vi "CG_Protokoll.vi"(6 "Aktion":T1, 8 "Pfad":path, 10 "Istwerte":dbl[](array[numeric]), 11 "Index":i32) -> (0 "Test läuft":bool, 1 "Abweichung":string[][](array[string]))   [LabVIEW 2020, in "Erweiterte Konfig.lvlib" / "CG-Check Konfig.lvlib"]
uses:
  CG-Check Konfig.lvlib
  Aktion_CG-Check_Protokoll.ctl
  Visualisierungs Elemente/String - Ausgabefeld.ctl
  Aktion_CG-Check.ctl
  FT-IR/FGV FT-IR Gasliste Aktionen.ctl
  Sprachverwaltung/FGV Aktion Tabelle zerlegen.ctl
  Schedule Modul/Aktion FGV Testdaten sammeln.ctl
  FT-IR/FT-IR.lvlib
  Schedule Modul/Schedule Modul.lvlib
  Sprachverwaltung/Sprachverwaltung.lvlib
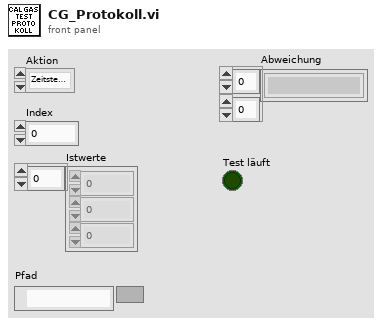
[diagram p1: front panel]
types:
  T1 = typedef "Erweiterte Konfig.lvlib/CG-Check Konfig.lvlib/Aktion_CG-Check_Protokoll.ctl" = enum16{"Zeitstempel", "Sollwerte", "Istwerte", "Vorzeitig beendet", "Auswerten", "Speichern", "Lesen"}
  T2 = typedef "String - Ausgabefeld.ctl" = string
  T3 = typedef "FT-IR.lvlib/FGV FT-IR Gasliste Aktionen.ctl" = enum16{"lesen", "Gasliste FT-IR", "Gasliste ausgelesen", "laden", "speichern", "löschen"}
  T4 = typedef "Erweiterte Konfig.lvlib/CG-Check Konfig.lvlib/Aktion_CG-Check.ctl" = enum16{"lesen", "schreiben", "laden", "Komponente", "Aktive?", "speichern"}
  T5 = typedef "Sprachverwaltung.lvlib/FGV Aktion Tabelle zerlegen.ctl" = enum16{"laden", "vereinzeln", "speichern"}
  T6 = typedef "Schedule Modul.lvlib/Aktion FGV Testdaten sammeln.ctl" = enum16{"lesen", "Dichtheitstest", "CalGasTest", "T90", "Kalibrieren", "init", "Kalender Daten"}
  T7 = enum16{"open", "replace", "create", "open or create", "replace or create", "replace or create with confirmation"}
  T8 = typedef "Schedule Modul.lvlib/Ergebnis CalGas Test.ctl" = cluster{"Istwerte":string[][], "Auswertung":string[][][], "Fehler":bool[], "Abweichung in %":string[][], "Spanauswahl":i32[]}
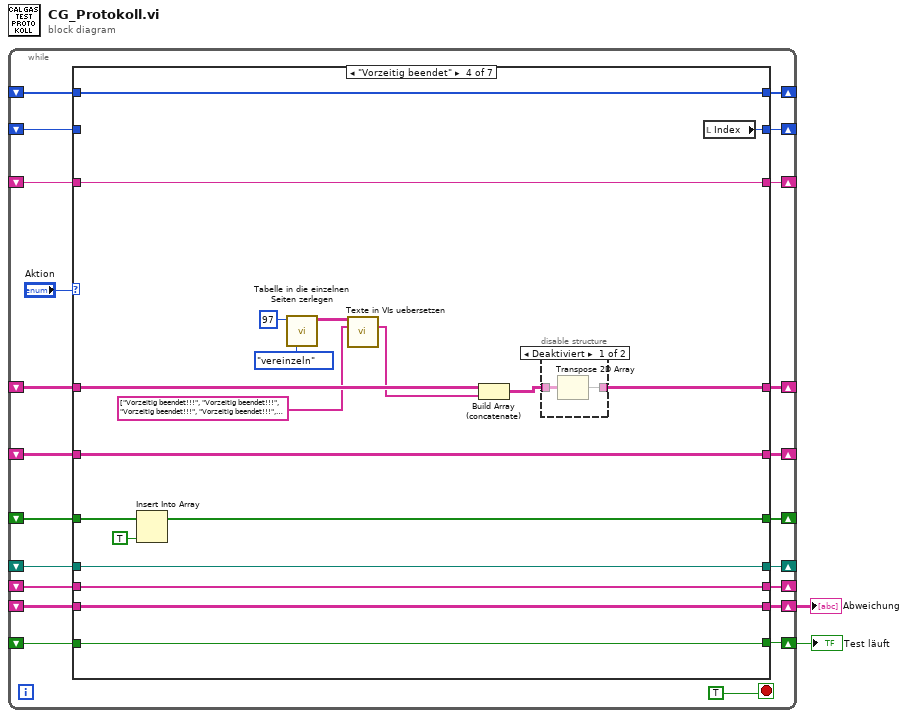
[diagram p0: block diagram]
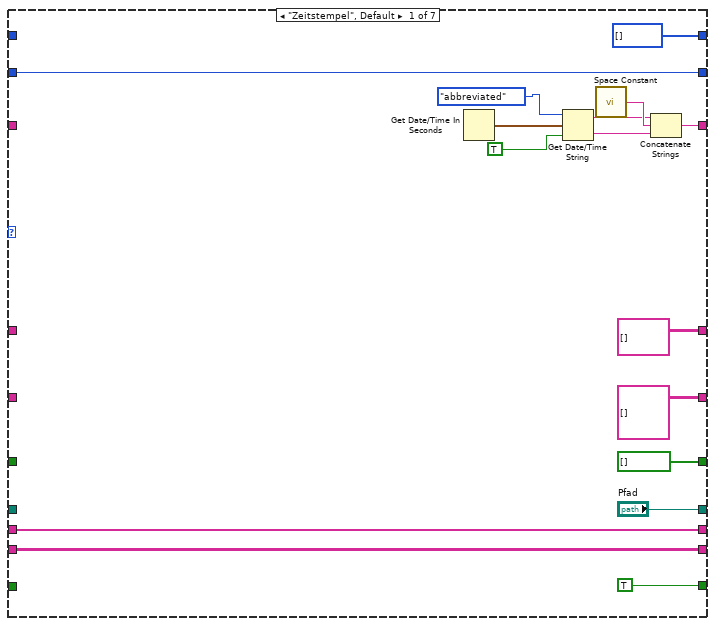
[diagram p2: hidden frame]
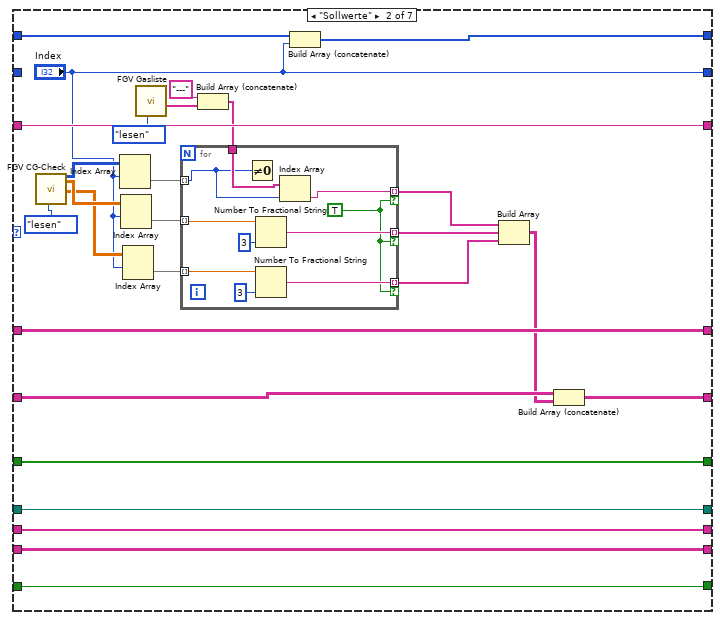
[diagram p3: hidden frame]
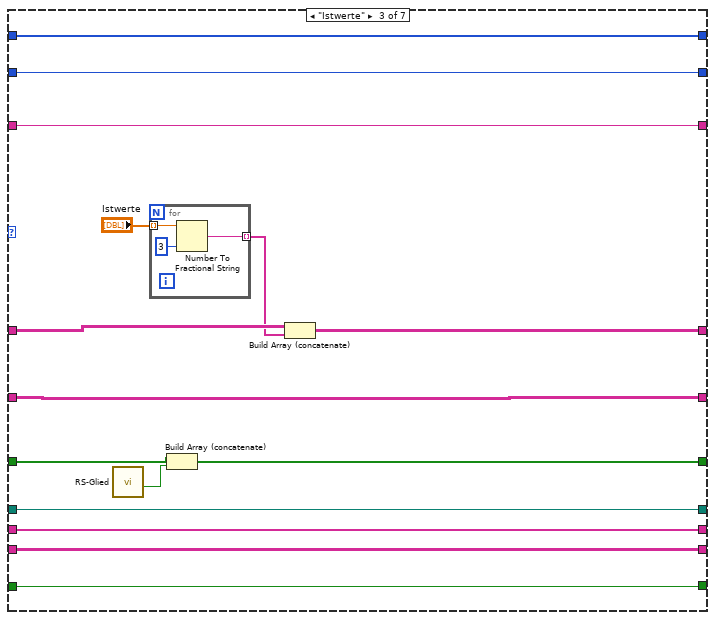
[diagram p4: hidden frame]
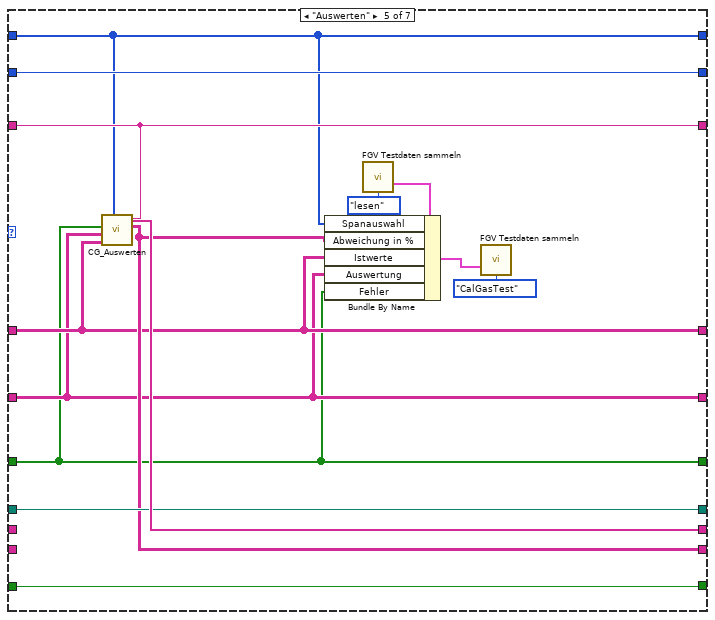
[diagram p6: hidden frame]
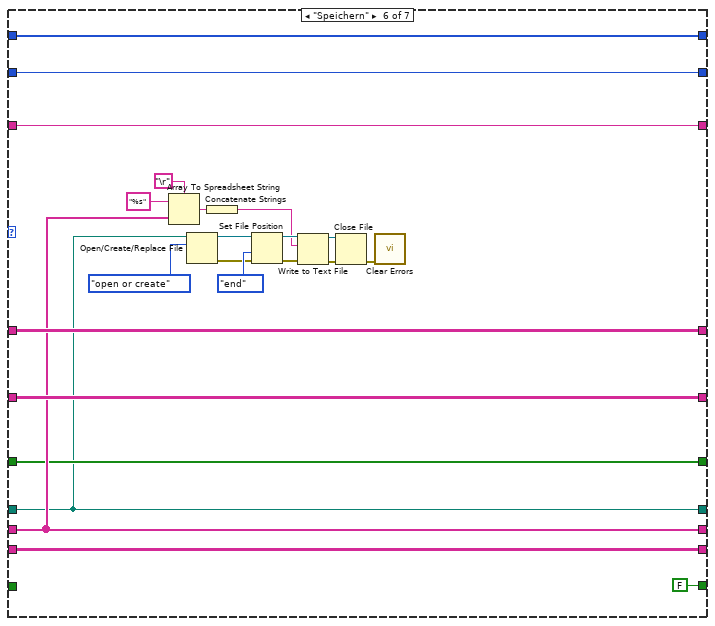
[diagram p7: hidden frame]
diagram:
  n1 = while {
    shift-right: [w23] -> _
    shift-left: _ -> [w22]
    shift-right: [w20] -> _
    shift-left: _ -> [w19]
    shift-right: [w18] -> _
    shift-left: _ -> [w17]
    shift-right: [w16] -> _
    shift-left: _ -> [w15]
    shift-right: [w14] -> _
    shift-left: _ -> [w13]
    shift-right: [w12] -> _
    shift-left: _ -> [w11]
    shift-right: [w10] -> _
    shift-left: _ -> [w9]
    shift-right: [w8] -> _
    shift-left: _ -> [w7]
    shift-right: [w6] -> w2
    shift-left: _ -> [w5]
    shift-right: [w4] -> w1
    shift-left: _ -> [w3]
    stop <- TRUE stop-if-true
    n2 = case shown="\"Vorzeitig beendet\"" "Aktion" {
      tunnel: [w34 w67 w91 w114 w128 w146 w164] -> w23
      tunnel: w22 -> [_ w67 w91 w114 w128 w146 w164]
      tunnel: [string[][] [] w59 w88 w111 w123 w154 w163] -> w20
      tunnel: w19 -> [_ w59 w90 w101 w123 w154 w163]
      tunnel: [T2[][][] [] w54 w89 w113 w122 w153 w162] -> w18
      tunnel: w17 -> [_ w55 w89 w113 w122 w153 w162]
      tunnel: [w31 "Index" w86 w105 w127 w145 w156] -> w16
      tunnel: w15 -> [w31 _ w86 _ w127 w145 w156]
      tunnel: [w33 w53 w87 w112 w131 w147 w161] -> w14
      tunnel: w13 -> [w33 w53 w87 w112 _ w147 w161]
      tunnel: [bool[] [] w52 w81 w108 w121 w144 w157] -> w12
      tunnel: w11 -> [_ w52 w80 w110 w121 w144 w157]
      tunnel: ["Pfad" w48 w85 w107 w130 w140 w160] -> w10
      tunnel: w9 -> [_ w48 w85 w107 w130 w140 w160]
      tunnel: [i32[] [] w44 w84 w106 w118 w137 w159] -> w8
      tunnel: w7 -> [_ w45 w84 w106 w118 w137 w159]
      tunnel: [TRUE w47 w83 w104 w129 FALSE w158] -> w6
      tunnel: w5 -> [_ w47 w83 w104 w129 _ w158]
      tunnel: [w29 w46 w82 w103 w124 w135 w155] -> w4
      tunnel: w3 -> [w29 w46 w82 w103 _ w135 w155]
      frame "Zeitstempel", Default {
        n3 = Get Date/Time In Seconds() -> (seconds since 1Jan1904=w35:timestamp)
        n4 = Get Date/Time String(date format (0)=enum16{"short", "long", "abbreviated"}."abbreviated" ("Datumsformat (0)"), seconds (now)=w35, want seconds? (F)=TRUE ("Angabe von Sekunden? (F)")) -> (date string=w38:string, time string=w40:string)
        n5 = call <vilib>:"Space Constant.vi"() -> ("String"=w39:string)
        n6 = Concatenate Strings(w38, w39, w40) -> (w34:string)
      }
      frame "Sollwerte" {
        n7 = call "FGV CG-Check.vi"("Aktion"=Aktion_CG-Check."lesen") -> ("Komponenten"=w65:u16[][], "Sollwerte"=w64:sgl[][], "max Abweichung"=w63:sgl[][])  [unwired: 11 in, 5 out]
        n8 = Index Array(array=w65, index (row)="Index") -> (element=w62:u16[])  [unwired: 1 in]
        n9 = Index Array(array=w64, index (row)="Index") -> (element=w61:sgl[])  [unwired: 1 in]
        n10 = Index Array(array=w63, index (row)="Index") -> (element=w60:sgl[])  [unwired: 1 in]
        n11 = call "FGV Gasliste.vi"("Aktionen"=FGV_FT-IR_Gasliste_Aktionen."lesen") -> ("Aktuelle Gasliste gesamt"=w51:T2[])  [unwired: 8 in, 2 out]
        n12 = Build Array (concatenate)("---", w51) -> (w50:T2[])
        n13 = for {
          tunnel: w62 -> [w72] mode=indexing
          tunnel: w61 -> [w77] mode=indexing
          tunnel: w60 -> [w75] mode=indexing
          tunnel: [w71] -> w58 mode=indexing if=w68
          tunnel: [w76] -> w57 mode=indexing if=w68
          tunnel: [w74] -> w56 mode=indexing if=w68
          tunnel: w50 -> [w73]
          w68 = TRUE
          n14 = Not Equal To 0?(x=w72) -> ()  [unwired: 1 out]
          n15 = Number To Fractional String(number=w77, precision (6)=i16 3 ("Genauigkeit (6)")) -> (F-format string=w76:string)  [unwired: 2 in]
          n16 = Number To Fractional String(number=w75, precision (6)=i16 3 ("Genauigkeit (6)")) -> (F-format string=w74:string)  [unwired: 2 in]
          n17 = Index Array(array=w73, index=w72) -> (element=w71:T2)
        }
        n18 = Build Array (concatenate)(w45, "Index") -> (w44:i32[])
        n19 = Build Array(w58, w57, w56) -> (w42:T2[][])
        n20 = Build Array (concatenate)(w55, w42) -> (w54:T2[][][])
      }
      frame "Istwerte" {
        n21 = call "RS-Glied.vi"() -> ("Fehler"=w79:bool)  [unwired: 11 in]
        n22 = for {
          tunnel: "Istwerte" -> [w95] mode=indexing
          tunnel: [w94] -> w78 mode=indexing
          n23 = Number To Fractional String(number=w95, precision (6)=i16 3 ("Genauigkeit (6)")) -> (F-format string=w94:string)  [unwired: 2 in]
        }
        n24 = Build Array (concatenate)(w80, w79) -> (w81:bool[])
        n25 = Build Array (concatenate)(w90, w78) -> (w88:string[][])
      }
      frame "Vorzeitig beendet" {
        n26 = Insert Into Array(array=w110, new element=TRUE ("Neues Element/Teil-Array")) -> (w108:bool[])  [unwired: 1 in]
        n27 = call "Tabelle in die einzelnen Seiten zerlegen.vi"("Aktion"=FGV_Aktion_Tabelle_zerlegen."vereinzeln", "Index (Seite)"=97) -> ("Sprachliste"=w97:string[][])  [unwired: 7 in, 2 out]
        n28 = call "Texte in VIs uebersetzen.vi"("Sprachliste"=w97, "String-Array zum Übersetzen"=string[] ["Vorzeitig beendet!!!", "Vorzeitig beendet!!!", "Vorzeitig beendet!!!", "Vorzeitig beendet!!!", "Vorzeitig beendet!!!"]) -> ("String-Array zum Übersetzen"=w96:string[])  [unwired: 9 in, 4 out]
        n29 = Build Array (concatenate)(w101, w96) -> (w102:string[][])
        n30 = disable-structure shown="Deaktiviert" {
          disable-tunnel: [w116 w117] -> w111
          disable-tunnel: w102 -> [w115 w117]
          frame Disabled {
            n31 = Transpose 2D Array(2D array=w115) -> (transposed array=w116:string[][])
          }
          frame Enabled {
          }
        }
        n32 = local read "Index"() -> (w105:i32)
      }
      frame "Auswerten" {
        n33 = call "CG_Auswerten.vi"("Span Auswahl"=w118, "Istwerte"=w123, "Sollwerte"=w122, "Fehler"=w121, "Zeitstempel"=w128) -> ("Abweichung"=w124:string[][], "Protokoll"=w131:string[])  [unwired: 5 in]
        n34 = call "FGV Testdaten sammeln.vi"("Aktion"=Aktion_FGV_Testdaten_sammeln."lesen") -> ("Ergebnis CalGas Test"=w125:T8)  [unwired: 9 in, 5 out]
        n35 = Bundle By Name(cluster=w125, "Spanauswahl"=w118, "Abweichung in %"=w124, "Istwerte"=w123, "Auswertung"=w122, "Fehler"=w121) -> (w120:T8)
        n36 = call "FGV Testdaten sammeln.vi"("Ergebnis CalGas Test"=w120, "Aktion"=Aktion_FGV_Testdaten_sammeln."CalGasTest") -> ()  [unwired: 8 in, 6 out]
      }
      frame "Speichern" {
        n37 = Array To Spreadsheet String(delimiter (Tab)="\r", array=w147, 3:"%s" ("Format-String")) -> (spreadsheet string=w132:string)
        n38 = Open/Create/Replace File(file path (use dialog)=w140, operation (0:open)=T7."open or create" ("Operation (0:Öffnen)")) -> (refnum out=w141:refnum<file>, error out=w142:errorcluster)  [unwired: 4 in, 1 out]
        n39 = Concatenate Strings(w132) -> (w134:string)
        n40 = Set File Position(refnum=w141, from (0:start)=enum16{"start", "end", "current"}."end" ("Von (0:Start)"), error in=w142) -> (refnum out=w139:refnum<file>, error out=w138:errorcluster)  [unwired: 1 in]
        n41 = Write to Text File(file (use dialog)=w139, text=w134, error in=w138) -> (refnum out=w151:refnum<file>, error out=w152:errorcluster)  [unwired: 1 in, 1 out]
        n42 = Close File(refnum=w151, error in=w152) -> (error out=w150:errorcluster)  [unwired: 1 out]
        n43 = call <vilib>:"Clear Errors.vi"("error in (no error)"=w150) -> ()  [unwired: 5 in, 2 out]
      }
      frame "Lesen" {
      }
    }
  }
  "Test läuft" <- w2
  "Abweichung" <- w1
